vi "Tetra_ADC_DRIVER.vi"(0 "COMPORT":refnum<visa-resource-name>="COM4", 11 "error in (no error)":errorcluster, 12 "EN_ADC_DRV":string(combo)="1", 13 "Open Ser(t)":bool, 14 "Close Ser(t)":bool) -> (2 "Success":bool=TRUE, 3 "output":string="rd reg 0x070 \r\n0x070: 0x0001\r\n>", 4 "comport":refnum<visa-resource-name>="COM4", 15 "error out":errorcluster)   [LabVIEW 2018]
panel:
  out "input 2":string
  out "output 2":string="rdiv\r\n0)  sw3p6:   195 mA  3616 mV\r\n1)  sw5p5:    89 mA  5472 mV\r\n2) sw2p8a:   315 mA  2784 mV\r\n3) sw2p8b:   349 mA  2768 mV\r\n4)  sw2p4:  1458 mA  2288 mV\r\n5)  sw1p4:  1047 mA  1304 mV\r\n>"
  out "input 1":string="rd reg 0x070 "
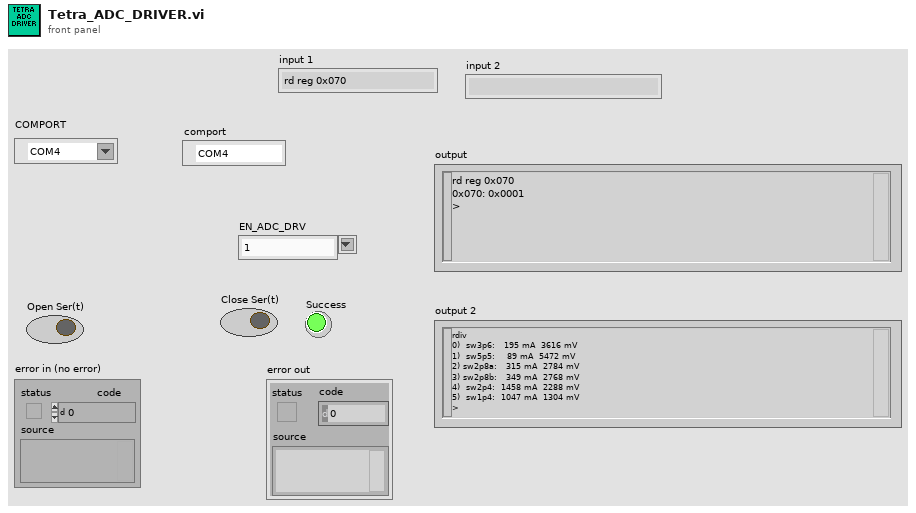
[diagram p1: front panel]
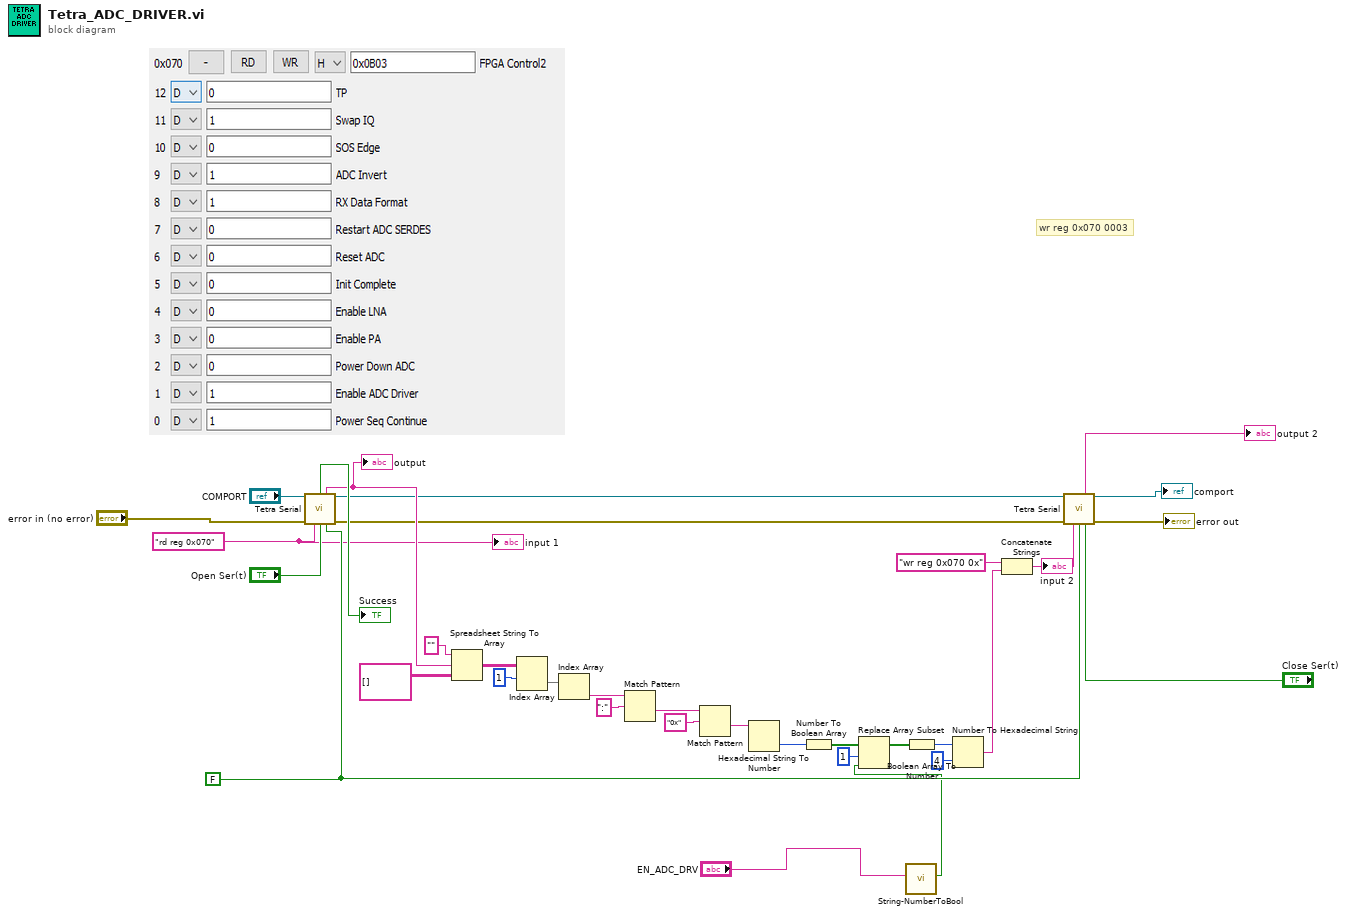
[diagram p0: block diagram]
diagram:
  w13 = FALSE ("Close Ser(t)")
  w7 = "rd reg 0x070" ("Command")
  # "wr reg 0x070 0003"
  n1 = call "Tetra Serial.vi"("COMPORT"="COMPORT", "error in (no error)"="error in (no error)", "Command"=w7, "Open Ser(t)"="Open Ser(t)", "Close Ser(t)"=w13) -> ("Success"=→"Success":bool, "output"=w30:string, "comport"=w15:refnum<visa-resource-name>, "error out"=w14:errorcluster)  [unwired: 6 in, 1 out]
  "output" <- w30
  n2 = Spreadsheet String To Array(format string="", spreadsheet string=w30, array type (2D Dbl)=string[][] []) -> (array=w27:string[][])  [unwired: 1 in]
  n3 = Index Array(array=w27, index (row)=1) -> (element=w25:string[])  [unwired: 1 in]
  n4 = Index Array(array=w25) -> (element=w24:string)  [unwired: 1 in]
  n5 = Match Pattern(string=w24, regular expression=":") -> (after substring=w22:string)  [unwired: 1 in, 3 out]
  n6 = Match Pattern(string=w22, regular expression="0x") -> (after substring=w20:string)  [unwired: 1 in, 3 out]
  n7 = Hexadecimal String To Number(string=w20) -> (number=w19:u32)  [unwired: 2 in, 1 out]
  n8 = Number To Boolean Array(number=w19) -> (Boolean array=w18:bool[])
  n9 = call "String-NumberToBool.vi"("String"="EN_ADC_DRV") -> ("Boolean"=w8:bool)  [unwired: 10 in]
  n10 = Replace Array Subset(array=w18, new element=w8, index=1) -> (w17:bool[])
  n11 = Boolean Array To Number(Boolean array=w17) -> (number=w16:u32)
  n12 = Number To Hexadecimal String(1:i16 4 ("width (-)"), 2:w16) -> (0:w12:string)
  n13 = Concatenate Strings("wr reg 0x070 0x" ("Command"), w12) -> (w4:string)
  "input 2" <- w4
  n14 = call "Tetra Serial.vi"("COMPORT"=w15, "error in (no error)"=w14, "Command"=w4, "Open Ser(t)"=w13, "Close Ser(t)"="Close Ser(t)") -> ("output"=→"output 2":string, "comport"=→"comport":refnum<visa-resource-name>, "error out"=→"error out":errorcluster)  [unwired: 6 in, 2 out]
  "input 1" <- w7
